vi "Serialize.vi"(8 "error in":errorcluster, 9 "OwningElement in":refnum<k20>, 10 "Document in":refnum<k20>, 11 "UserComment in":refnum<class "UserComment.lvclass">) -> (0 "error out":errorcluster, 1 "OwningElement out":refnum<k20>, 2 "Document out":refnum<k20>, 3 "UserComment out":refnum<class "UserComment.lvclass">)   [LabVIEW 2021, in "ProligentXMLGenerator.lvlib" / "UserComment.lvclass"]
uses:
  UserComment.lvclass
  UserComment.lvclass/UserComment.ctl
  Base/DOMSupport/DOMSupport.lvlib
  <vilib>/xml/NI_XML.lvlib
  <vilib>/xml/Close Reference(Node).vi
  Base/DateTime/DateTime.lvclass
  C:/Projects/proligent-xml-generator-labview/src/ProligentXMLGenerator/Base/Attribute/Attribute.lvclass
  C:/Projects/proligent-xml-generator-labview/src/ProligentXMLGenerator/Base/DateTime/DateTime.lvclass
  Base/NonEmptyString_255/NonEmptyString_255.lvclass
  C:/Projects/proligent-xml-generator-labview/src/ProligentXMLGenerator/Base/NonEmptyString/NonEmptyString.lvclass
  C:/Projects/proligent-xml-generator-labview/src/ProligentXMLGenerator/Base/String/String.lvclass
  C:/Projects/proligent-xml-generator-labview/src/ProligentXMLGenerator/Base/NonEmptyString_255/NonEmptyString_255.lvclass
  Base/NonNullableString_TruncateAt_255/NonNullableString_TruncateAt_255.lvclass
  C:/Projects/proligent-xml-generator-labview/src/ProligentXMLGenerator/Base/NonNullableString/NonNullableString.lvclass
  C:/Projects/proligent-xml-generator-labview/src/ProligentXMLGenerator/Base/NonNullableString_TruncateAt_255/NonNullableString_TruncateAt_255.lvclass
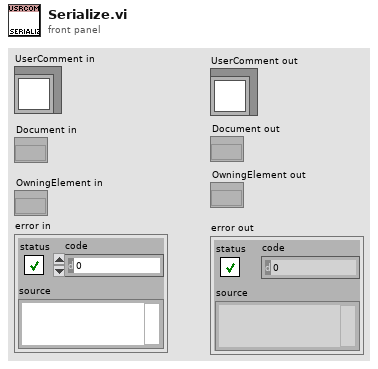
[diagram p1: front panel]
types:
  T1 = typedef "ProligentXMLGenerator.lvlib/UserComment.lvclass/Data.ctl" = cluster{"Name":string, "Comment":refnum<class "NonNullableString_TruncateAt_255.lvclass">, "User":refnum<class "NonEmptyString_255.lvclass">, "Time":refnum<class "DateTime.lvclass">}
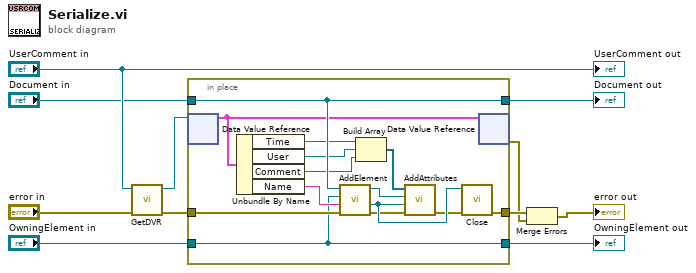
[diagram p0: block diagram]
diagram:
  n1 = call "GetDVR.vi"("error in"="error in", "UserComment"="UserComment in") -> ("error out"=w3:errorcluster, "DVRReference"=w2:refnum<data-value>)  [unwired: 8 in]
  n2 = in-place "In Place Element Structure" {
    in-place-border: [w23] -> w4
    in-place-border: "Document in" -> [w22]
    in-place-border: w3 -> [w25]
    in-place-border: "OwningElement in" -> [w21]
    in-place-border: [w22] -> w6
    in-place-border: [w21] -> w5
    n3 = in-place-dvr #1(w2) -> (w20:T1)  [unwired: 1 out]
    n4 = Unbundle By Name(w20) -> ("Time"=w19:refnum<class "DateTime.lvclass">, "User"=w18:refnum<class "NonEmptyString_255.lvclass">, "Comment"=w17:refnum<class "NonNullableString_TruncateAt_255.lvclass">, "Name"=w24:string)
    n5 = call "AddElement.vi"("error in"=w25, "Name"=w24, "OwningElement in"=w21, "Document in"=w22) -> ("error out"=w12:errorcluster, "NewElement"=w15:refnum<k20>, "Document out"=w14:refnum<k20>)  [unwired: 4 in, 1 out]
    n6 = Build Array(w19, w18, w17) -> (w16:refnum<class "Attribute.lvclass">[])
    n7 = call "AddAttributes.vi"("error in"=w12, "OwningElement in"=w15, "Document in"=w14, "Attributes"=w16) -> ("error out"=w13:errorcluster)  [unwired: 5 in, 2 out]
    n8 = call-poly <vilib>:"Close.vi"("error in (no error)"=w13, "node"=w15) -> ("error out"=w23:errorcluster)  [unwired: 7 in]
    n9 = in-place-dvr #1(w20) -> (w1:errorcluster)  [unwired: 1 out]
  }
  "OwningElement out" <- w5
  "Document out" <- w6
  n10 = Merge Errors(w4, w1) -> (→"error out":errorcluster)
  "UserComment out" <- "UserComment in"
